vi "CtrlMain.vi"   [LabVIEW 2016]
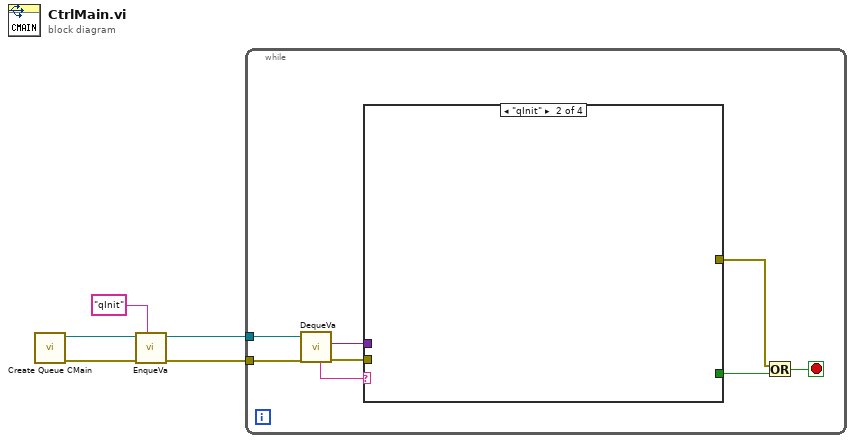
[diagram p0: block diagram]
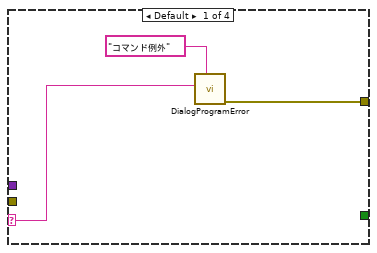
[diagram p2: hidden frame]
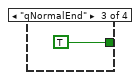
[diagram p3: hidden frame]
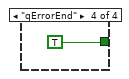
[diagram p4: hidden frame]
diagram:
  n1 = call "Create Queue CMain.vi"() -> ("error out"=w3:errorcluster, "queCMain"=w5:refnum<queue>)  [unwired: 10 in]
  n2 = call "EnqueVa.vi"("コマンド"="qInit", "エラー入力（エラーなし）"=w3, "queVariant"=w5) -> ("エラー出力"=w2:errorcluster, "queVariant(copy)"=w4:refnum<queue>)  [unwired: 6 in, 1 out]
  n3 = while {
    tunnel: w2 -> [w13]
    tunnel: w4 -> [w12]
    stop <- w6 stop-if-true
    n4 = call "DequeVa.vi"("エラー入力（エラーなし）"=w13, "queVariant"=w12) -> ("エラー出力"=w10:errorcluster, "バリアント"=w9:variant, "コマンド"=w11:string)  [unwired: 5 in, 2 out]
    n5 = case shown="\"qInit\"" w11 {
      selector: w11 -> [w15 _ _ _]
      tunnel: w10 -> [_ _ _ _]
      tunnel: w9 -> [_ _ _ _]
      tunnel: [w14 _ _ _] -> w8
      tunnel: [_ _ TRUE TRUE] -> w7
      frame Default {
        n6 = call "DialogProgramError.vi"("エラー内容"="コマンド例外", "エラー詳細"=w15) -> ("error out"=w14:errorcluster)  [unwired: 9 in]
      }
      frame "qInit" {
      }
      frame "qNormalEnd" {
      }
      frame "qErrorEnd" {
      }
    }
    n7 = Or(x=w8, y=w7) -> (x .or. y?=w6:bool)
  }
